vi "FHSLidar_video_back_subst.vi"() -> ()   [LabVIEW 2020]
uses:
  <vilib>/userdefined/High Color/IMAQdx.ctl
  <vilib>/Analysis/baseanly.llb/Mean (DBL).vi
  <resource>/objmgr/imaqdx.rc
  <vilib>/vision/driver/NI_Vision_Acquisition_Software.lvlib
  <vilib>/Analysis/NI_AALBase.lvlib
panel:
  in  "Display wavelength end":dbl=50.0
  in  "Chlorophyll end":dbl=50.0
  in  "Powder end":dbl=54.0
  in  "Elastic  end":dbl=60.0
  in  "Use single wavelength (off=ROI)":bool
  out "loop number":i32
  in  "nbr_im":i32=10
  in  "Background substraction":bool
  in  "Display wavelength start":dbl=50.0
  out "Frame Rate":dbl
  out "write info file":bool
  out "range time":dbl[][](graph)
  out "RGB int range":dbl[][](graph)
  in  "Powder start":dbl=54.0
  in  "Chlorophyll start":dbl=50.0
  in  "Elastic start":dbl=60.0
  out "Intensity \nwavelength":i16[](graph)
  out "Intensity Graph":i16[][](graph)
  out "error out 2":errorcluster
  in  "Binning Spect":dbl=1.0
  in  "Binning Range":dbl=2.0
  in  "File Path Control":path
  in  "Gain<=24":dbl=24.0
  out "error out":errorcluster
  in  "Exposure time (us)":dbl=8000.0
  in  "Cancel Button":bool
  in  "OK Button":bool
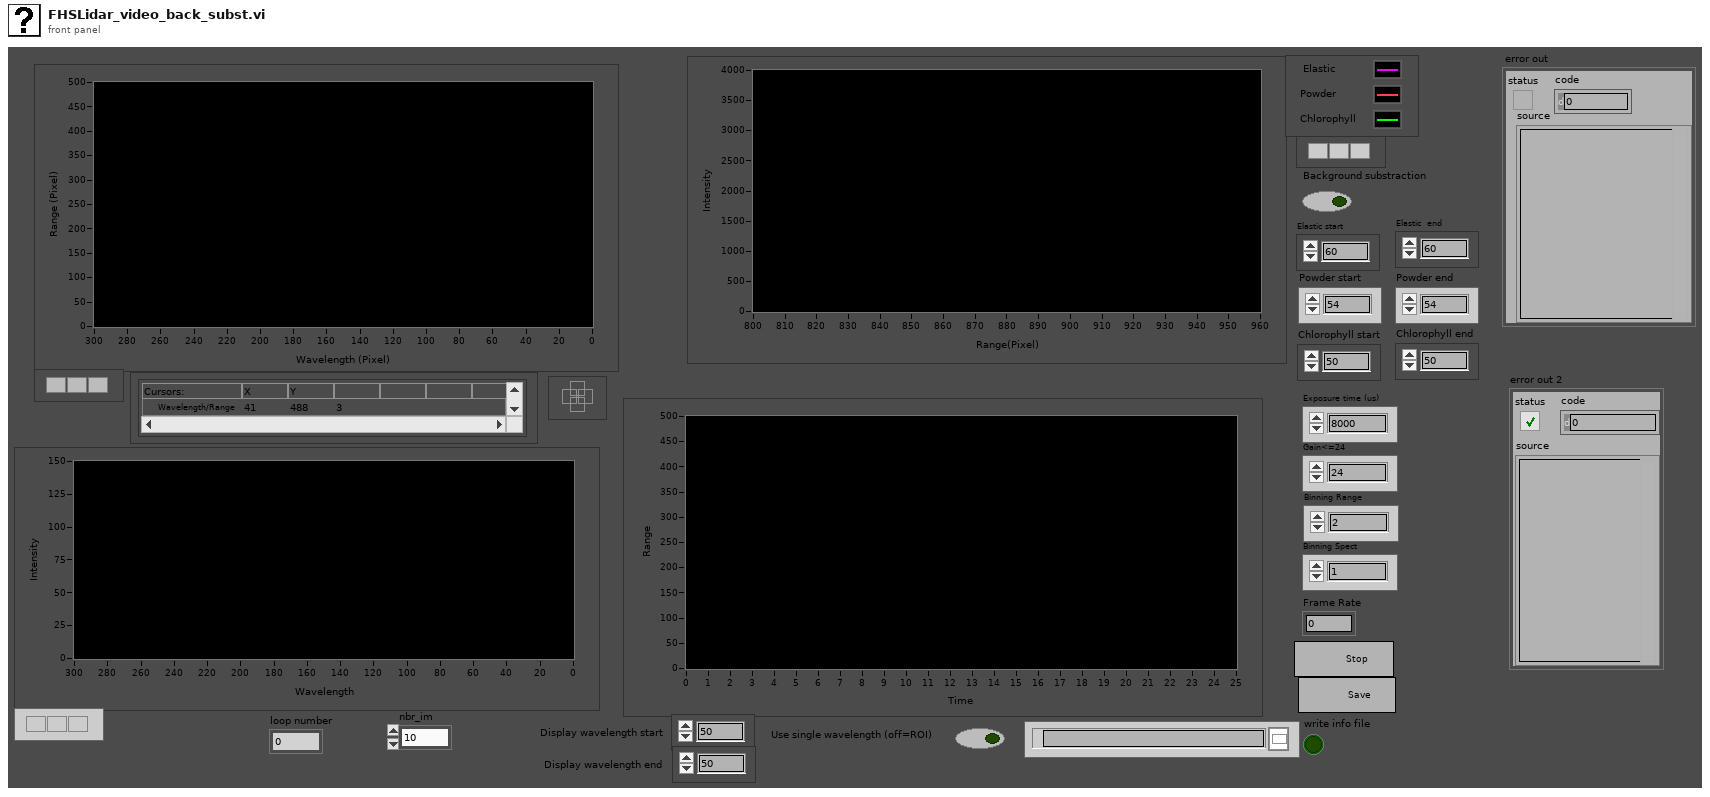
[diagram p1: front panel]
types:
  T1 = typedef "IMAQdx.ctl" = refnum<k21>
  T2 = typedef "IMAQ Image.ctl" = refnum<image>
  T3 = enum16{"open", "replace", "create", "open or create", "replace or create", "replace or create with confirmation"}
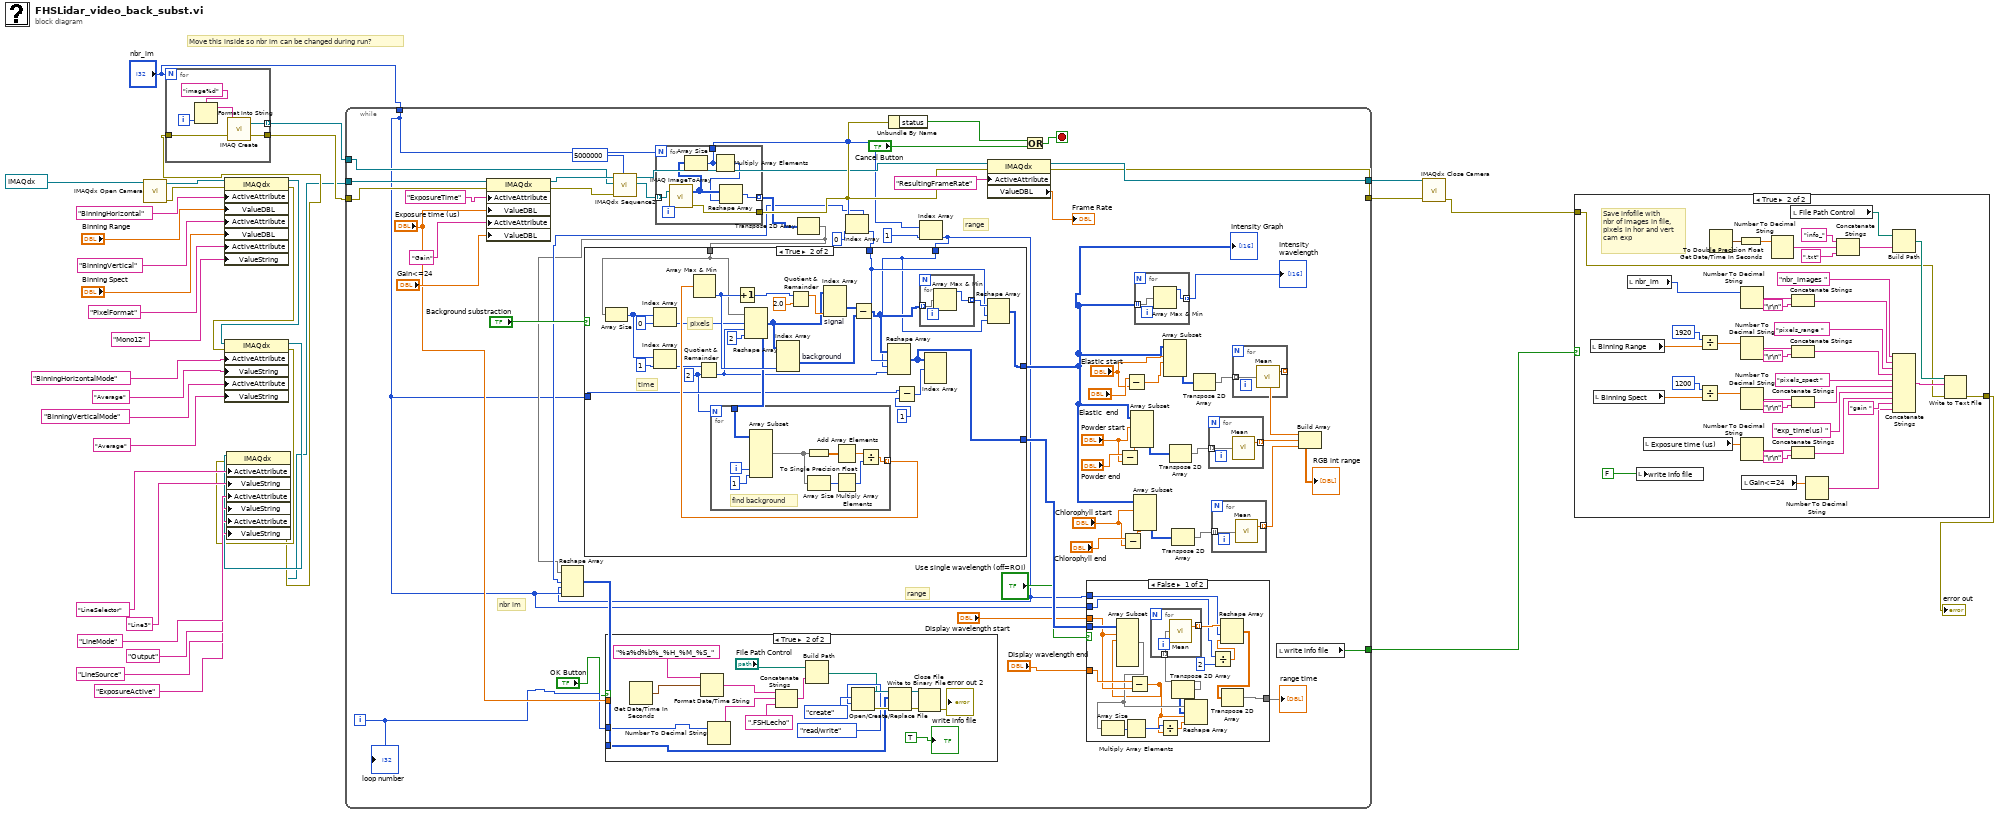
[diagram p0: block diagram]
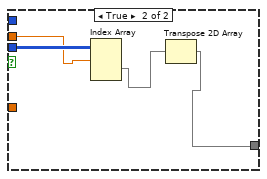
[diagram p3: hidden frame]
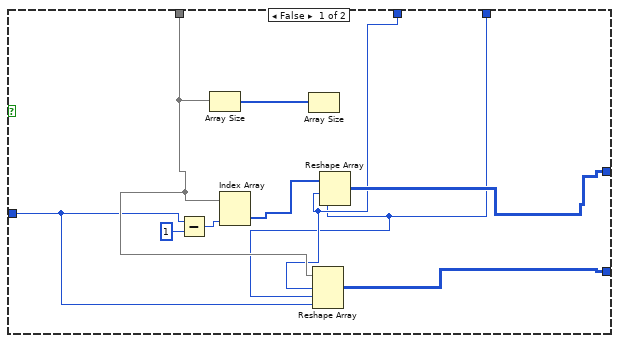
[diagram p4: hidden frame]
diagram:
  # "Move this inside so nbr im can be changed during run?"
  n1 = call <vilib>:"IMAQdx Open Camera.vi"("Session In"=T1 "cam1") -> ("error out"=w6:errorcluster, "Session Out"=w27:T1)  [unwired: 9 in]
  n2 = property class="IMAQdx"(reference=w27, error in=w6, "ActiveAttribute"="BinningHorizontal", "ValueDBL"="Binning Range", "ActiveAttribute"="BinningVertical", "ValueDBL"="Binning Spect", "ActiveAttribute"="PixelFormat", "ValueString"="Mono12") -> (reference out=w16:T1, error out=w15:errorcluster)
  n3 = property class="IMAQdx"(reference=w16, error in=w15, "ActiveAttribute"="BinningHorizontalMode", "ValueString"="Average" ("ActiveAttribute"), "ActiveAttribute"="BinningVerticalMode", "ValueString"="Average" ("ActiveAttribute")) -> (reference out=w8:T1, error out=w7:errorcluster)
  n4 = property class="IMAQdx"(reference=w8, error in=w7, "ActiveAttribute"="LineSelector", "ValueString"="Line3" ("ActiveAttribute"), "ActiveAttribute"="LineMode", "ValueString"="Output" ("ActiveAttribute"), "ActiveAttribute"="LineSource", "ValueString"="ExposureActive" ("ActiveAttribute")) -> (reference out=w3:T1, error out=w5:errorcluster)
  n5 = for {
    N: "nbr_im" -> [_]
    tunnel: w5 -> [w39]
    tunnel: [w38] -> w2 mode=indexing
    tunnel: [w37] -> w4
    i -> [w36]
    n6 = Format Into String(format string="image%d" ("Image Name"), w36) -> (resulting string=w35:string)  [unwired: 2 in, 1 out]
    n7 = call "IMAQ Create"("Image Name"=w35, "error in (no error)"=w39) -> ("New Image"=w38:T2, "error out"=w37:errorcluster)  [unwired: 2 in, 1 out]
  }
  n8 = while {
    tunnel: w3 -> [w98]
    tunnel: w2 -> [w80]
    tunnel: w4 -> [w97]
    tunnel: [w86] -> w33
    tunnel: [w85] -> w32
    tunnel: [w90] -> w21
    tunnel: "nbr_im" -> [w42]
    i -> [w83]
    stop <- w94 stop-if-true
    # "range"
    # "nbr im"
    # "range"
    n9 = property class="IMAQdx"(reference=w98, error in=w97, "ActiveAttribute"="ExposureTime", "ValueDBL"="Exposure time (us)", "ActiveAttribute"="Gain", "ValueDBL"="Gain<=24") -> (reference out=w81:T1, error out=w82:errorcluster)
    n10 = call <vilib>:"IMAQdx Sequence2.vi"("Timeout (ms)"=5000000, "error in"=w82, "Images In"=w80, "Session In"=w81) -> ("Images Out"=w78:T2[], "Session Out"=w79:T1)  [unwired: 5 in, 1 out]
    n11 = for {
      N: w42 -> [_]
      tunnel: [w200] -> w87
      tunnel: [w196] -> w72 mode=indexing
      tunnel: w78 -> [w199] mode=indexing
      tunnel: [w195] -> w71
      n12 = call "IMAQ ImageToArray"("Image"=w199) -> ("error out"=w200:errorcluster, "Image Pixels (I16)"=w198:i16[][])  [unwired: 3 in, 3 out]
      n13 = Array Size(array=w198) -> (size(s)=w195:i32[])
      n14 = Multiply Array Elements(1:w195) -> (0:w197:i32)
      n15 = Reshape Array(w198, w197) -> (w196:i16[])
    }
    n16 = Transpose 2D Array(2D array=w72) -> (transposed array=w65:i16[][])
    n17 = Index Array(array=w71, index=0) -> (element=w66:i32)
    n18 = Unbundle By Name(w87) -> ("status"=w96:bool)
    n19 = Index Array(array=w71, index=1) -> (element=w41:i32)
    n20 = Reshape Array(w65, w66, w41, w42) -> (w64:i16[][][])
    n21 = case shown="True" "Background substraction" {
      tunnel: w65 -> [w134 w148]
      tunnel: [w135 w140] -> w45
      tunnel: w42 -> [w131 w151]
      tunnel: [w130 w152] -> w73
      tunnel: w66 -> [w133 w142]
      tunnel: w41 -> [w132 w141]
      frame False {
        n22 = Subtract(x=w131, y=1) -> (x-y=w137:i32)
        n23 = Array Size(array=w134) -> (size(s)=w138:i32[])
        n24 = Index Array(array=w134, index (col)=w137) -> (element=w136:i16[])  [unwired: 1 in]
        n25 = Array Size(array=w138) -> ()  [unwired: 1 out]
        n26 = Reshape Array(w134, w133, w132, w131) -> (w130:i16[][][])
        n27 = Reshape Array(w136, w133, w132) -> (w135:i16[][])
      }
      frame True {
        w150 = 2 ("dimension size")
        # "time"
        # "pixels"
        n28 = Array Size(array=w148) -> (size(s)=w164:i32[])
        n29 = Index Array(array=w164, index=0) -> (element=w147:i32)
        n30 = Index Array(array=w164, index=1) -> (element=w146:i32)
        n31 = Quotient & Remainder(x=w146, y=w150) -> (floor(x/y)=w145:i32)  [unwired: 1 out]
        n32 = Reshape Array(w148, w147, w145, 2 ("dimension size")) -> (w156:i16[][][])
        n33 = for {
          N: w150 -> [_]
          tunnel: [w175] -> w161 mode=indexing
          tunnel: w156 -> [w170]
          i -> [w172]
          # "find background"
          n34 = Array Subset(array=w170, index (dim 2)=w172, length (dim 2)=1 ("intervals")) -> (w169:i16[][][])  [unwired: 4 in]
          n35 = To Single Precision Float(number=w169) -> (single precision float=w168:sgl[][][])
          n36 = Array Size(array=w169) -> (size(s)=w173:i32[])
          n37 = Add Array Elements(numeric array=w168) -> (sum=w174:sgl)
          n38 = Multiply Array Elements(1:w173) -> (0:w176:i32)
          n39 = Divide(x=w174, y=w176) -> (x/y=w175:sgl)
        }
        n40 = Array Max & Min(array=w161) -> (min index (indices)=w158:i32)  [unwired: 3 out]
        n41 = Increment(x=w158) -> (x+1=w160:i32)
        n42 = Index Array "background"(array=w156, index (dim 2)=w158) -> (element=w149:i16[][])  [unwired: 2 in]
        n43 = Quotient & Remainder(x=w160, y=2.0) -> (x-y*floor(x/y)=w157:dbl)  [unwired: 1 out]
        n44 = Index Array "signal"(array=w156, index (dim 2)=w157) -> (element=w155:i16[][])  [unwired: 2 in]
        n45 = Subtract(x=w155, y=w149) -> (x-y=w144:i16[][])
        n46 = Reshape Array(w144, w142, w141, w145) -> (w152:i16[][][])
        n47 = Subtract(x=w151, y=1) -> (x-y=w153:i32)
        n48 = for {
          tunnel: [w166] -> w143 mode=indexing
          tunnel: w144 -> [w167] mode=indexing
          n49 = Array Max & Min(array=w167) -> (max value=w166:i16)  [unwired: 3 out]
        }
        n50 = Index Array(array=w152, index (dim 0)=w153) -> ()  [unwired: 2 in, 1 out]
        n51 = Reshape Array(w143, w142, w141) -> (w140:i16[][])
      }
    }
    "Intensity Graph" <- w45
    n52 = case shown="True" "OK Button" {
      tunnel: "Exposure time (us)" -> [_ _]
      tunnel: w83 -> [_ w178]
      tunnel: w64 -> [_ w182]
      frame False {
      }
      frame True {
        n53 = Get Date/Time In Seconds() -> (seconds since 1Jan1904=w180:timestamp)
        n54 = Format Date/Time String(time format string (%c)="%a%d%b%_%H_%M_%S_", seconds (now)=w180) -> (date/time string=w177:string)  [unwired: 1 in]
        n55 = Number To Decimal String(number=w178) -> (decimal integer string=w183:string)  [unwired: 1 in]
        n56 = Concatenate Strings(w177, w183, ".FSHLecho" ("string")) -> (w187:string)
        n57 = Build Path(base path="File Path Control", name or relative path=w187) -> (appended path=w184:path)
        n58 = Open/Create/Replace File(file path (use dialog)=w184, operation (0:open)=T3."create", access (0:read/write)=enum16{"read/write", "read-only", "write-only"}."read/write") -> (refnum out=w194:refnum<file>, error out=w191:errorcluster)  [unwired: 3 in, 1 out]
        n59 = Write to Binary File(file (use dialog)=w194, data=w182, error in=w191) -> (refnum out=w193:refnum<file>, error out=w192:errorcluster)  [unwired: 3 in, 1 out]
        n60 = Close File(refnum=w193, error in=w192) -> (error out=→"error out 2":errorcluster)  [unwired: 1 out]
        "write info file" <- TRUE
      }
    }
    n61 = property class="IMAQdx"(reference=w79, error in=w87, "ActiveAttribute"="ResultingFrameRate") -> (reference out=w86:T1, error out=w85:errorcluster, "ValueDBL"=→"Frame Rate":dbl)
    n62 = Or(x=w96, y="Cancel Button") -> (x .or. y?=w94:bool)
    n63 = case shown="False" "Use single wavelength (off=ROI)" {
      tunnel: w73 -> [w120 w127]
      tunnel: "Display wavelength start" -> [w119 w126]
      tunnel: [w118 w124] -> w67
      tunnel: "Display wavelength end" -> [w121 _]
      tunnel: w42 -> [w107 _]
      tunnel: w41 -> [w108 _]
      frame False {
        n64 = Subtract(x=w121, y=w119) -> (x-y=w113:dbl)
        n65 = Array Subset(array=w120, index (dim 0)=w119, length (dim 0)=w113) -> (w117:i16[][][])  [unwired: 4 in]
        n66 = Array Size(array=w117) -> (size(s)=w116:i32[])
        n67 = Multiply Array Elements(1:w116) -> (0:w115:i32)
        n68 = Divide(x=w115, y=w113) -> (x/y=w114:dbl)
        n69 = Reshape Array(w117, w113, w114) -> (w112:i16[][])
        n70 = Transpose 2D Array(2D array=w112) -> (transposed array=w111:i16[][])
        n71 = for {
          tunnel: w111 -> [w123] mode=indexing
          tunnel: [w122] -> w110 mode=indexing
          n72 = call-poly <vilib>:"Mean.vi"("X"=w123) -> ("mean"=w122:dbl)  [unwired: 1 out]
        }
        n73 = Divide(x=w107, y=2) -> (x/y=w105:dbl)
        n74 = Reshape Array(w110, w108, w105) -> (w109:dbl[][])
        n75 = Transpose 2D Array(2D array=w109) -> (transposed array=w118:dbl[][])
      }
      frame True {
        n76 = Index Array(array=w127, index (dim 0)=w126) -> (element=w125:i16[][])  [unwired: 2 in]
        n77 = Transpose 2D Array(2D array=w125) -> (transposed array=w124:i16[][])
      }
    }
    "range time" <- w67
    n78 = Subtract(x="Powder end", y="Powder start") -> (x-y=w52:dbl)
    n79 = Subtract(x="Chlorophyll end", y="Chlorophyll start") -> (x-y=w48:dbl)
    n80 = Subtract(x="Elastic  end", y="Elastic start") -> (x-y=w61:dbl)
    n81 = Array Subset(array=w45, index (row)="Powder start", length (row)=w52) -> (w56:i16[][])  [unwired: 2 in]
    n82 = Array Subset(array=w45, index (row)="Chlorophyll start", length (row)=w48) -> (w50:i16[][])  [unwired: 2 in]
    n83 = for {
      tunnel: [w128] -> w74 mode=indexing
      tunnel: w45 -> [w129] mode=indexing
      n84 = Array Max & Min(array=w129) -> (max value=w128:i16)  [unwired: 3 out]
    }
    "Intensity \nwavelength" <- w74
    n85 = Array Subset(array=w45, index (row)="Elastic start", length (row)=w61) -> (w58:i16[][])  [unwired: 2 in]
    n86 = Transpose 2D Array(2D array=w56) -> (transposed array=w55:i16[][])
    n87 = Transpose 2D Array(2D array=w50) -> (transposed array=w49:i16[][])
    n88 = Transpose 2D Array(2D array=w58) -> (transposed array=w57:i16[][])
    n89 = for {
      tunnel: [w102] -> w51 mode=indexing
      tunnel: w55 -> [w101] mode=indexing
      n90 = call-poly <vilib>:"Mean.vi"("X"=w101) -> ("mean"=w102:dbl)  [unwired: 1 out]
    }
    n91 = for {
      tunnel: [w100] -> w44 mode=indexing
      tunnel: w49 -> [w99] mode=indexing
      n92 = call-poly <vilib>:"Mean.vi"("X"=w99) -> ("mean"=w100:dbl)  [unwired: 1 out]
    }
    n93 = for {
      tunnel: [w104] -> w62 mode=indexing
      tunnel: w57 -> [w103] mode=indexing
      n94 = call-poly <vilib>:"Mean.vi"("X"=w103) -> ("mean"=w104:dbl)  [unwired: 1 out]
    }
    n95 = local read "write info file"() -> (w90:bool)
    n96 = Build Array(w62, w51, w44) -> (→"RGB int range":dbl[][])
    "loop number" <- w83
  }
  n97 = call <vilib>:"IMAQdx Close Camera.vi"("error in"=w32, "Session In"=w33) -> ("error out"=w23:errorcluster)  [unwired: 9 in]
  n98 = case shown="True" w21 {
    tunnel: w23 -> [w201 w205]
    tunnel: [w201 w204] -> w22
    frame False {
    }
    frame True {
      # "Save infofile with\nnbr of images in file,\npixels in hor and vert\ncam exp"
      n99 = local read "Binning Range"() -> (w237:dbl)
      n100 = local read "Binning Spect"() -> (w233:dbl)
      n101 = local read "nbr_im"() -> (w202:i32)
      n102 = local write "write info file"(FALSE) -> ()
      n103 = local read "Exposure time (us)"() -> (w230:dbl)
      n104 = Divide(x=1920, y=w237) -> (x/y=w236:dbl)
      n105 = Divide(x=1200, y=w233) -> (x/y=w232:dbl)
      n106 = Get Date/Time In Seconds() -> (seconds since 1Jan1904=w227:timestamp)
      n107 = To Double Precision Float(number=w227) -> (double precision float=w228:dbl)
      n108 = Number To Decimal String(number=w202) -> (decimal integer string=w213:string)  [unwired: 1 in]
      n109 = Number To Decimal String(number=w236) -> (decimal integer string=w215:string)  [unwired: 1 in]
      n110 = Number To Decimal String(number=w232) -> (decimal integer string=w217:string)  [unwired: 1 in]
      n111 = Number To Decimal String(number=w230) -> (decimal integer string=w210:string)  [unwired: 1 in]
      n112 = local read "Gain<=24"() -> (w208:dbl)
      n113 = Number To Decimal String(number=w228) -> (decimal integer string=w226:string)  [unwired: 1 in]
      n114 = local read "File Path Control"() -> (w223:path)
      n115 = Concatenate Strings(w213, "\r\n") -> (w212:string)
      n116 = Concatenate Strings(w215, "\r\n") -> (w214:string)
      n117 = Concatenate Strings(w217, "\r\n") -> (w216:string)
      n118 = Concatenate Strings(w210, "\r\n") -> (w209:string)
      n119 = Number To Decimal String(number=w208) -> (decimal integer string=w206:string)  [unwired: 1 in]
      n120 = Concatenate Strings("info_" ("string"), w226, ".txt" ("string")) -> (w222:string)
      n121 = Build Path(base path=w223, name or relative path=w222) -> (appended path=w221:path)
      n122 = Concatenate Strings("nbr_images " ("ActiveAttribute"), w212, "pixels_range " ("ActiveAttribute"), w214, "pixels_spect ", w216, "exp_time(us) " ("ActiveAttribute"), w209, "gain " ("ActiveAttribute"), w206) -> (w229:string)
      n123 = Write to Text File(file (use dialog)=w221, text=w229, error in=w205) -> (error out=w204:errorcluster)  [unwired: 1 in, 2 out]
    }
  }
  "error out" <- w22
